vi "Thermistor_Temperature.vi"(1 "T word":u16) -> (0 "Temperature (degC)":sgl=25.0)   [LabVIEW 2015]
panel:
  in  "T0 (K)":sgl=298.15
  in  "R1(T0) (ohms)":sgl=100000.0
  in  "R2 (ohms)":sgl=100000.0
  in  "B (K)":sgl=4250.0
  in  "Vs (V)":sgl=3.3
  # "Paul Nathan 26/07/2012"
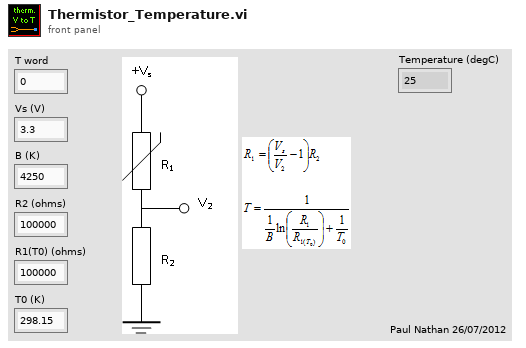
[diagram p1: front panel]
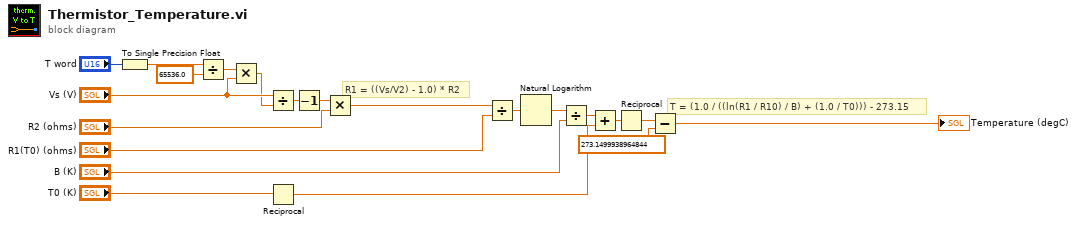
[diagram p0: block diagram]
diagram:
  # "T = (1.0 / ((ln(R1 / R10) / B) + (1.0 / T0))) - 273.15"
  # "R1 = ((Vs/V2) - 1.0) * R2"
  n1 = To Single Precision Float(number="T word") -> (single precision float=w5:sgl)
  n2 = Divide(x=w5, y=sgl 65536.0) -> (x/y=w4:sgl)
  n3 = Multiply(x=w4, y="Vs (V)") -> (x*y=w1:sgl)
  n4 = Divide(x="Vs (V)", y=w1) -> (x/y=w21:sgl)
  n5 = Reciprocal(x="T0 (K)") -> (1/x=w14:sgl)
  n6 = Decrement(x=w21) -> (x-1=w19:sgl)
  n7 = Multiply(x=w19, y="R2 (ohms)") -> (x*y=w18:sgl)
  n8 = Divide(x=w18, y="R1(T0) (ohms)") -> (x/y=w12:sgl)
  n9 = Natural Logarithm(1:w12) -> (0:w11:sgl)
  n10 = Divide(x=w11, y="B (K)") -> (x/y=w10:sgl)
  n11 = Add(x=w10, y=w14) -> (x+y=w9:sgl)
  n12 = Reciprocal(x=w9) -> (1/x=w8:sgl)
  n13 = Subtract(x=w8, y=sgl 273.15) -> (x-y=→"Temperature (degC)":sgl)
